vi "Check ref frame has been selected (simple).vi"(8 "error in (no error)":errorcluster) -> (0 "error out":errorcluster, 3 "Proceed / Reference frame has been selected":bool)   [LabVIEW 2020]
uses:
  Typedefs/Set Main VI cursor.ctl
  Global Variables/General Globals.vi
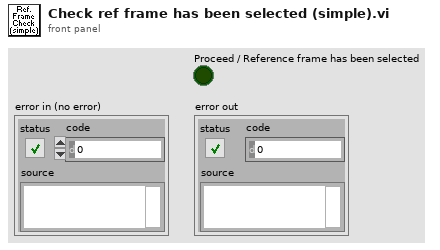
[diagram p1: front panel]
types:
  T1 = typedef "Set Main VI cursor.ctl" = enum16{"Release busy cursor", "Set busy cursor"}
  T2 = typedef "Reference_Globals.ctl" = cluster{"Refrence data path":path, "Reference Rectangle":i16[][], "AOL Z":dbl, "No of pixels in a miniscan ":i32[], "Threshold":i16[], "No of miniscans":i32[], "Full Frame Size":u16, "Reference Image":T3, "dwelltime":dbl, "Zoom":dbl, "Field of View":dbl, "Z Step":i8, "Z pixels":i32, "Z Lines":u8, "Z Ignore":u8, "Laser":u8}
  T3 = typedef "IMAQ Image.ctl" = refnum<image>
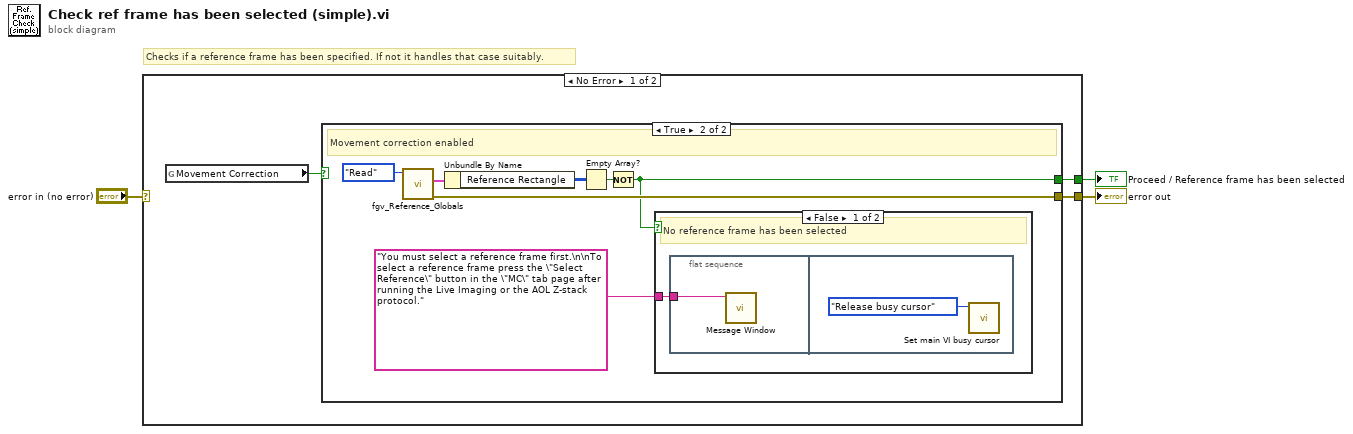
[diagram p0: block diagram]
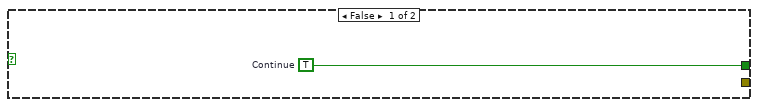
[diagram p2: hidden frame]
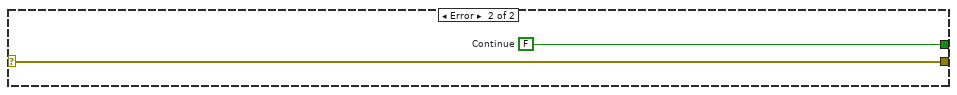
[diagram p4: hidden frame]
diagram:
  # "Checks if a reference frame has been specified. If not it handles that case suitably."
  n1 = case shown="No Error" "error in (no error)" {
    selector: "error in (no error)" -> [_ w19]
    tunnel: [w6 w18] -> w3
    tunnel: [w4 w19] -> w1
    frame No Error {
      n2 = global read "General Globals.vi" "Movement Correction"() -> (w5:bool)
      n3 = case shown="True" w5 {
        tunnel: [w7 w9] -> w6
        tunnel: [_ w10] -> w4
        frame False {
          w7 = TRUE  # Continue
        }
        frame True {
          # "Movement correction enabled"
          n4 = call "fgv_Reference_Globals.vi"("Function"=enum16{"Intialize", "Write", "Read", "Clear"}."Read") -> ("error out"=w10:errorcluster, "Reference Data"=w13:T2)  [unwired: 9 in]
          n5 = Unbundle By Name(w13) -> ("Reference Rectangle"=w12:i16[][])
          n6 = Empty Array?(array=w12) -> (empty?=w11:bool)
          n7 = Not(x=w11) -> (.not. x?=w9:bool)
          n8 = case shown="False" w9 {
            tunnel: "You must select a reference frame first.\n\nTo select a reference frame press the \"Select Reference\" button in the \"MC\" tab page after running the Live Imaging or the AOL Z-stack protocol." ("Message string") -> [w15 _]
            frame False {
              # "No reference frame has been selected"
              n9 = flat-sequence {
                tunnel: w15 -> [w16]
                frame #0 {
                  n10 = call "Message Window.vi"("Message string"=w16) -> ()  [unwired: 10 in, 1 out]
                }
                frame #1 {
                  n11 = call "Set main VI busy cursor.vi"("Main VI's cursor"=Set_Main_VI_cursor."Release busy cursor") -> ()  [unwired: 10 in, 1 out]
                }
              }
            }
            frame True {
              # "Reference frame has been selected"
            }
          }
        }
      }
    }
    frame Error {
      w18 = FALSE  # Continue
    }
  }
  "Proceed / Reference frame has been selected" <- w3
  "error out" <- w1
